vi "Fields Query.vi"(6 "Return Data? (T)":bool=TRUE, 8 "error in (no error)":errorcluster, 10 "Query":string, 11 "Connection Refnum":T4) -> (0 "error out":errorcluster, 2 "Fields":T1[](array[typedef]), 3 "Connection Refnum":T4, 4 "Data Present?":bool)   [LabVIEW 2011]
uses:
  Summitek/Win32/ODBC/SQL Controls/Connection Refnum.ctl
  typedefs/Field Record.ctl
  typedefs/Field DataTypes.ctl
  typedefs/Field NextItem.ctl
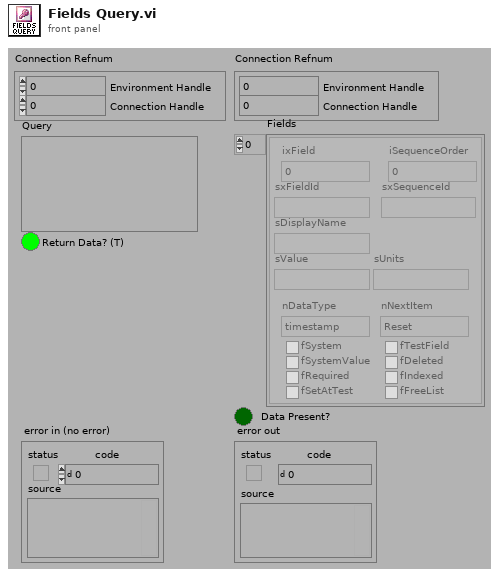
[diagram p1: front panel]
types:
  T1 = typedef "Field Record.ctl" = cluster{"ixField":i32, "iSequenceOrder":i32, "sxFieldId":string, "sxSequenceId":string, "sDisplayName":string, "sValue":string, "sUnits":string, "nDataType":T2, "nNextItem":T3, "fSystem":bool, "fSystemValue":bool, "fRequired":bool, "fSetAtTest":bool, "fTestField":bool, "fDeleted":bool, "fIndexed":bool, "fFreeList":bool}
  T2 = typedef "Field DataTypes.ctl" = enum32{"text", "numeric", "list", "timestamp", "boolean"}
  T3 = typedef "Field NextItem.ctl" = enum32{"Reset", "Retain", "Auto-Increment"}
  T4 = typedef "Connection Refnum.ctl" = cluster{"Environment Handle":i32, "Connection Handle":i32}
  T5 = typedef "Statement Refnum.ctl" = cluster{"Statement Handle":i32, "Parameter Number":u16}
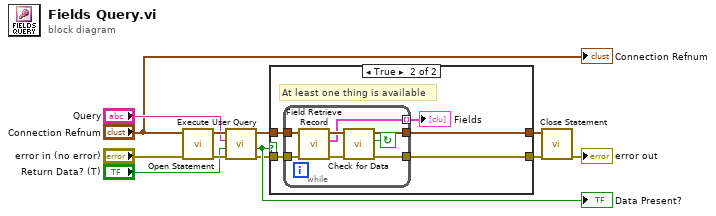
[diagram p0: block diagram]
diagram:
  n1 = call "Open Statement.vi"("error in (no error)"="error in (no error)", "Connection Refnum"="Connection Refnum") -> ("error out"=w8:errorcluster, "Statement Refnum"=w9:T5)  [unwired: 4 out]
  n2 = call "Execute User Query.vi"("error in (no error)"=w8, "Return Data? (f)"="Return Data? (T)", "User Query"="Query", "Statement Refnum"=w9) -> ("error out"=w11:errorcluster, "Data Present?"=w12:bool, "Statement Refnum"=w10:T5)  [unwired: 1 out]
  "Data Present?" <- w12
  n3 = case shown="True" w12 {
    tunnel: w11 -> [w13 w18]
    tunnel: w10 -> [w14 w19]
    tunnel: [w13 w15] -> w7
    tunnel: [w14 w17] -> w6
    frame False {
      # "Query Returned no matching fields."
    }
    frame True {
      # "At least one thing is available"
      n4 = while {
        tunnel: w19 -> [w26]
        tunnel: w18 -> [w25]
        tunnel: [w23] -> w17
        tunnel: [w21] -> w15
        tunnel: [w20] -> w16 mode=indexing
        stop <- w27 continue-if-true
        n5 = call "Field Retrieve Record.vi"("error in (no error)"=w25, "Statement Refnum"=w26) -> ("error out"=w22:errorcluster, "Field Record"=w20:T1, "Statement Refnum"=w24:T5)  [unwired: 7 out]
        n6 = call "Check for Data.vi"("error in (no error)"=w22, "Statement Refnum"=w24) -> ("error out"=w21:errorcluster, "Data Present?"=w27:bool, "Statement Refnum"=w23:T5)  [unwired: 3 out]
      }
      "Fields" <- w16
    }
  }
  n7 = call "Close Statement.vi"("error in (no error)"=w7, "Statement Refnum"=w6) -> ("error out"=→"error out":errorcluster)  [unwired: 5 out]
  "Connection Refnum" <- "Connection Refnum"
